vi "PPG_ABC.check config.vi"(0 "i ref in":refnum<vi>, 2 "PGData":T1, 5 "error in (no error)":errorcluster) -> (14 "i ref out":refnum<vi>, 16 "PGData out":T1, 19 "error out":errorcluster)   [LabVIEW 2014, in "PPG_ABC.lvlib"]
doc: "Checks, if the configuration is reasonable."
uses:
  PPG_ABC.lvlib
  PPG_ABC.PG_dataType.ctl
  CSCore/CSSystem/CoreDefs/CoreDefs.error_type.ctl
  CSCore/CSSystem/CoreDefs/CoreDefs.error_severity.ctl
  CSCore/CSSystem/CoreLib/CoreLib.lvlib
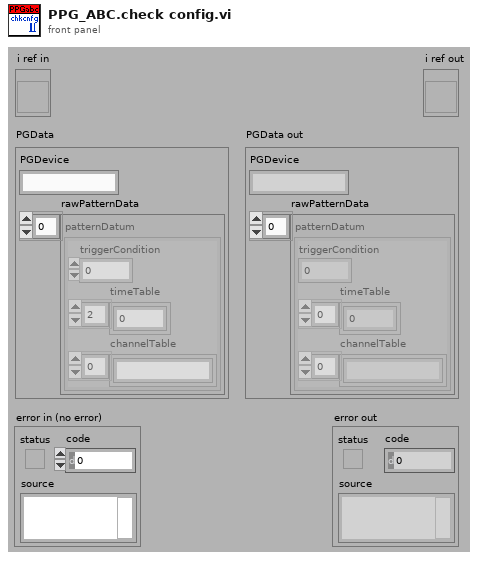
[diagram p1: front panel]
types:
  T1 = typedef "PPG_ABC.lvlib/PPG_ABC.PG_dataType.ctl" = cluster{"PGDevice":string, "rawPatternData":cluster{"triggerCondition":i32, "timeTable":dbl[], "channelTable":string[]}[]}
  T2 = typedef "CoreDefs.error_severity.ctl" = enum16{"undefined", "information", "warning", "error", "fatal"}
  T3 = typedef "CoreDefs.error_type.ctl" = enum16{"no error", "can't load process", "can't unload process", "process does not exist", "can't install process", "can't remove process", "unknown function", "time out", "can't execute function", "duplicate queue name", "super not found", "caller queue invalid", "can't ping process", "unknown error", "VISA Error", "VISA timeout", "GPIB timeout", "GPIB error", "communication error", "data type mismatch", "can't read data from OPC server", "can't write data to OPC server", "OET error", "function not implemented", "process already exists", "invalid Shared Variable name", "error writing Shared Variable", "error reading Shared Variable", "invalid client name", "corrupt database", "unknown class", "call not authorized", "parameter out of range", "OET timeout: can't get data to modify", "invalid queue name", "requested operation incompatible with current state", "event undefined", "event disabled", "state undefined", "caller is not a friend", "EventBuilder: bad eventID", "EventBuilder: no DAQ devices", "a thread must not stop itself", "UNUSED ELEMENT4", "DiscArchiver: eventData incomplete", "DiscArchiver: eventData does not belong to run", "DiscArchiver: can't open file", "DiscArchiver: can't write to file", "DiscArchiver: available disc space low", "can't acquire semaphore", "error reading data from database", "notifier object is not existing", "can't register process", "can't unregister process", "illegal event type", "object disabled", "object already exists", "can't change state", "Instrument not found", "no connection to remote node", "invalid reference", "N/A", "UNUSED ELEMENT 1", "element not found", "illegal TCP/IP connection detected", "object does not exist", "invalid access ID", "unknown CS system", "invalid privilige", "unsupported data type", "unsupported server type", "IO server already exists", "Shared Variable already exists"}
  T4 = cluster{"triggerCondition":i32, "timeTable":dbl[], "channelTable":string[]}[]
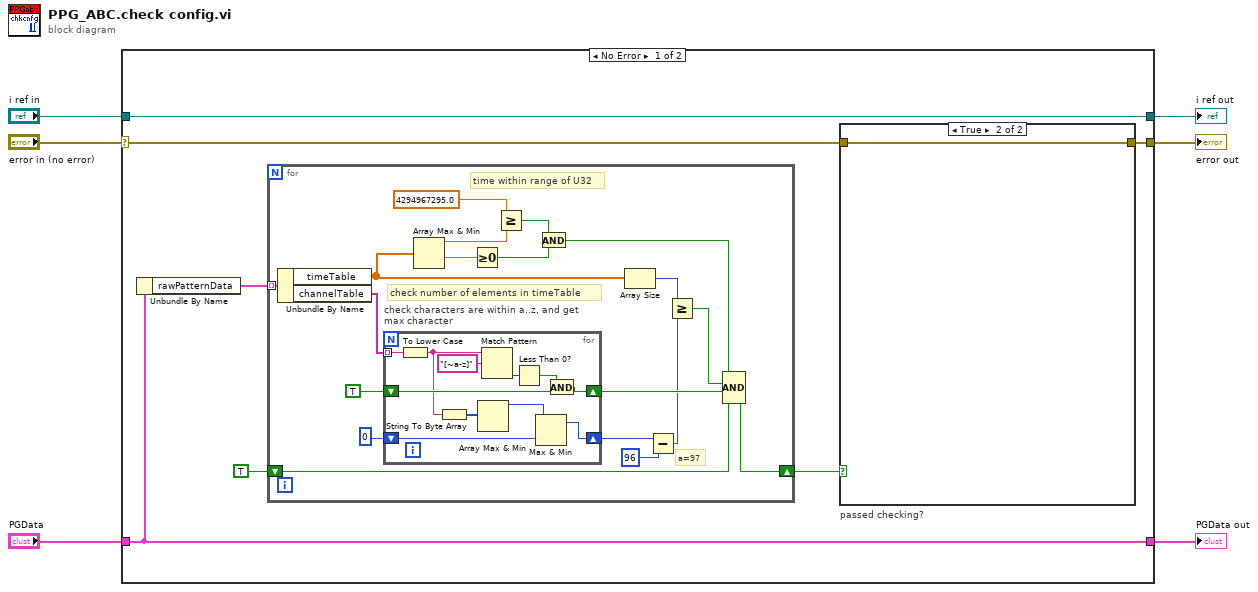
[diagram p0: block diagram]
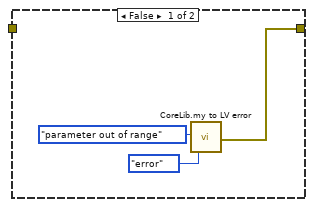
[diagram p2: hidden frame]
diagram:
  n1 = case shown="No Error" "error in (no error)" {
    selector: "error in (no error)" -> [w9 w48]
    tunnel: "i ref in" -> [w13 w49]
    tunnel: [w13 w49] -> w5
    tunnel: [w8 w48] -> w4
    tunnel: [w7 _] -> w2
    tunnel: "PGData" -> [w7 _]
    frame No Error {
      n2 = Unbundle By Name(w7) -> ("rawPatternData"=w12:T4)
      n3 = for {
        tunnel: w12 -> [w36] mode=indexing
        shift-right: [w27] -> w10
        shift-left: TRUE -> [w28]
        # "a=97"
        # "check number of elements in timeTable"
        # "time within range of U32"
        n4 = Unbundle By Name(w36) -> ("timeTable"=w25:dbl[], "channelTable"=w31:string[])
        n5 = for "check characters are within a..z, and get\nmax character" {
          tunnel: w31 -> [w46] mode=indexing
          shift-right: [w42] -> w29
          shift-left: TRUE -> [w43]
          shift-right: [w37] -> w21
          shift-left: 0 -> [w39]
          n6 = To Lower Case(string=w46) -> (all lower case string=w41:string)
          n7 = String To Byte Array(string=w41) -> (unsigned byte array=w40:u8[])
          n8 = Array Max & Min(array=w40) -> (max value=w38:u8)  [unwired: 3 out]
          n9 = Match Pattern(string=w41, regular expression="[~a-z]") -> (offset past match=w45:i32)  [unwired: 1 in, 3 out]
          n10 = Less Than 0?(x=w45) -> (x < 0?=w44:bool)
          n11 = Max & Min(x=w38, y=w39) -> (max(x,y)=w37:i32)  [unwired: 1 out]
          n12 = And(x=w44, y=w43) -> (x .and. y?=w42:bool)
        }
        n13 = Array Max & Min(array=w25) -> (max value=w18:dbl, min value=w35:dbl)  [unwired: 2 out]
        n14 = Greater Or Equal To 0?(x=w35) -> (x >= 0?=w33:bool)
        n15 = Greater Or Equal?(x=4294967295.0, y=w18) -> (x >= y?=w32:bool)
        n16 = And(x=w32, y=w33) -> (x .and. y?=w22:bool)
        n17 = Array Size(array=w25) -> (size(s)=w24:i32)
        n18 = Subtract(x=w21, y=96) -> (x-y=w19:i32)
        n19 = Greater Or Equal?(x=w24, y=w19) -> (x >= y?=w23:bool)
        n20 = Compound Arithmetic op=AND(w22, w23, w29, w28) -> (w27:bool)
      }
      n21 = case "passed checking?" shown="True" w10 {
        tunnel: w9 -> [_ w17]
        tunnel: [w15 w17] -> w8
        frame False {
          n22 = call "CoreLib.my to LV error.vi"("ErrorTypes"=CoreDefs.error_type."parameter out of range", "severityLevel"=CoreDefs.error_severity."error") -> ("myErrorCluster"=w15:errorcluster)  [unwired: 16 in, 1 out]
        }
        frame True {
        }
      }
    }
    frame Error {
    }
  }
  "error out" <- w4
  "i ref out" <- w5
  "PGData out" <- w2
